vi "Lex Open Delimiter.vi"(8 "Error In":errorcluster, 11 "Lexer In":refnum<class "Lexer.lvclass">) -> (0 "Error Out":errorcluster, 3 "Lexer Out":refnum<class "Lexer.lvclass">)   [LabVIEW 2018, in "Toolkit.lvlib" / "Lexer.lvclass"]
uses:
  Lexer.lvclass
  Lexer.lvclass/Lexer.ctl
  States.ctl
  Tokens/Text/Text.lvclass
  D:/Users/cfield/Code/Field R&D Services/Labstache/src/Toolkit/Low-Level/Tokens/Token/Token.lvclass
  Tokens/Text/New.vi
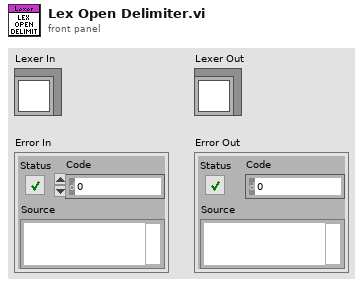
[diagram p1: front panel]
types:
  T1 = typedef "Toolkit.lvlib/Lexer.lvclass/States.ctl" = enum16{"Text", "Open Delimiter", "Tag Type", "Tag Key", "Close Delimiter"}
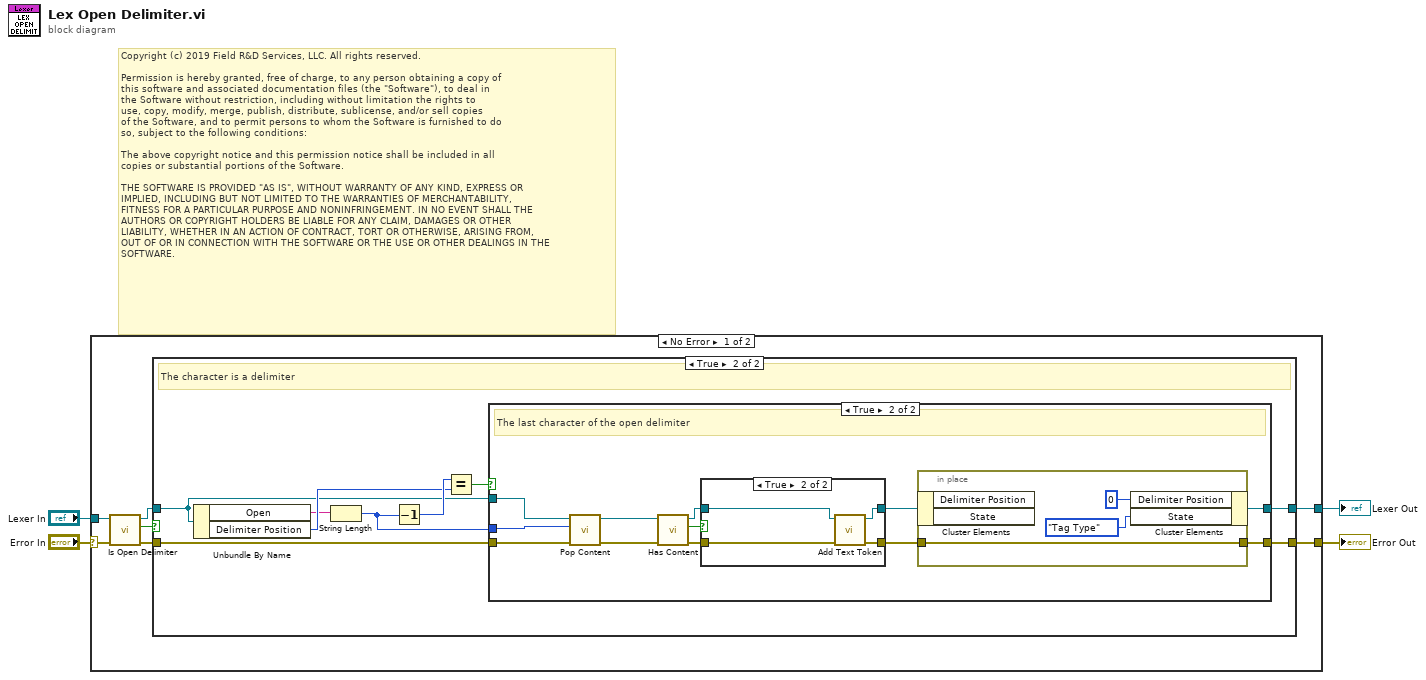
[diagram p0: block diagram]
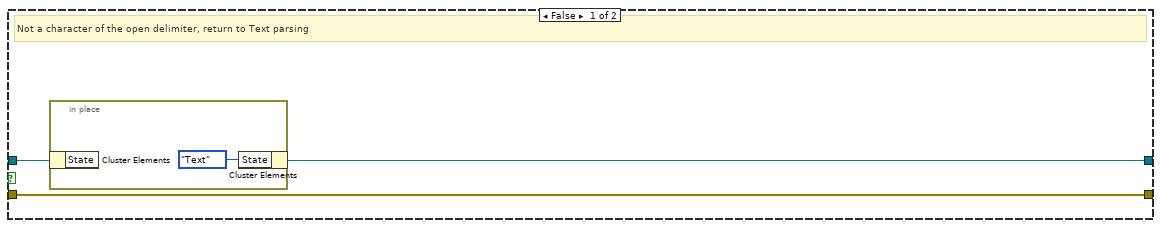
[diagram p2: hidden frame]
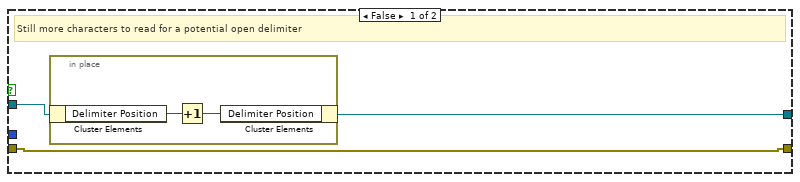
[diagram p3: hidden frame]
diagram:
  # "Copyright (c) 2019 Field R&D Services, LLC. All rights reserved.\n\nPermission is hereby granted, free of charge, to any person obtaining a copy of\nthis software and associated documentation files (the \"Software\"), to deal in\nthe Software without restriction, including without limitation the rights to\nuse, copy, modify, merge, publish, distribute, sublicense, and/or sell copies\nof the Software, and to permit persons to whom the Software is furnished to do\nso, subject to the following conditions:\n\nThe above copyright notice and this permission notice shall be included in all\ncopies or substantial portions of the Software.\n\nTHE SOFTWARE IS PROVIDED \"AS IS\", WITHOUT WARRANTY OF ANY KIND, EXPRESS OR\nIMPLIED, INCLUDING BUT NOT LIMITED TO THE WARRANTIES OF MERCHANTABILITY,\nFITNESS FOR A PARTICULAR PURPOSE AND NONINFRINGEMENT. IN NO EVENT SHALL THE\nAUTHORS OR COPYRIGHT HOLDERS BE LIABLE FOR ANY CLAIM, DAMAGES OR OTHER\nLIABILITY, WHETHER IN AN ACTION OF CONTRACT, TORT OR OTHERWISE, ARISING FROM,\nOUT OF OR IN CONNECTION WITH THE SOFTWARE OR THE USE OR OTHER DEALINGS IN THE\nSOFTWARE."
  n1 = case shown="No Error" "Error In" {
    selector: "Error In" -> [w10 w51]
    tunnel: [w6 w51] -> w4
    tunnel: [w5 w52] -> w3
    tunnel: "Lexer In" -> [w11 w52]
    frame No Error {
      n2 = call "Is Open Delimiter.vi"("Error In"=w10, "Lexer In"=w11) -> ("Error Out"=w9:errorcluster, "Open Delimiter"=w7:bool, "Lexer Out"=w8:refnum<class "Lexer.lvclass">)  [unwired: 7 in]
      n3 = case shown="True" w7 {
        tunnel: w9 -> [w14 w21]
        tunnel: w8 -> [w13 w20]
        tunnel: [w14 w18] -> w6
        tunnel: [w12 w19] -> w5
        frame False {
          # "Not a character of the open delimiter, return to Text parsing"
          n4 = in-place {
            n5 = in-place-cluster #1(w13) -> ()  [unwired: 1 out]
            n6 = in-place-cluster #1("State"=States."Text") -> (w12:refnum<class "Lexer.lvclass">)
          }
        }
        frame True {
          # "The character is a delimiter"
          n7 = Unbundle By Name(w20) -> ("Open"=w17:string, "Delimiter Position"=w23:i32)
          n8 = String Length(string=w17) -> (length=w16:i32)
          n9 = Decrement(x=w16) -> (x-1=w24:i32)
          n10 = Equal?(x=w24, y=w23) -> (x = y?=w22:bool)
          n11 = case shown="True" w22 {
            tunnel: w21 -> [w25 w40]
            tunnel: w20 -> [w27 w41]
            tunnel: [w26 w34] -> w19
            tunnel: [w25 w35] -> w18
            tunnel: w16 -> [_ w39]
            frame False {
              # "Still more characters to read for a potential open delimiter"
              n12 = in-place {
                n13 = in-place-cluster #2(w27) -> ("Delimiter Position"=w29:i32)
                n14 = Increment(x=w29) -> (x+1=w28:i32)
                n15 = in-place-cluster #2("Delimiter Position"=w28) -> (w26:refnum<class "Lexer.lvclass">)
              }
            }
            frame True {
              # "The last character of the open delimiter"
              n16 = call "Pop Content.vi"("Error In"=w40, "Characters Count"=w39, "Lexer In"=w41) -> ("Error Out"=w32:errorcluster, "Lexer Out"=w38:refnum<class "Lexer.lvclass">)  [unwired: 7 in]
              n17 = call "Has Content.vi"("Error In"=w32, "Lexer In"=w38) -> ("Error Out"=w31:errorcluster, "Content"=w30:bool, "Lexer Out"=w33:refnum<class "Lexer.lvclass">)  [unwired: 7 in]
              n18 = case shown="True" w30 {
                tunnel: [w43 w47] -> w37
                tunnel: [w42 w46] -> w36
                tunnel: w33 -> [w43 w45]
                tunnel: w31 -> [w42 w44]
                frame False {
                }
                frame True {
                  n19 = call "Add Text Token.vi"("Error In"=w44, "Lexer In"=w45) -> ("Error Out"=w46:errorcluster, "Lexer Out"=w47:refnum<class "Lexer.lvclass">)  [unwired: 8 in]
                }
              }
              n20 = in-place {
                in-place-border: w36 -> [w50]
                in-place-border: [w50] -> w35
                n21 = in-place-cluster #3(w37) -> ()  [unwired: 2 out]
                n22 = in-place-cluster #3("Delimiter Position"=0, "State"=States."Tag Type") -> (w34:refnum<class "Lexer.lvclass">)
              }
            }
          }
        }
      }
    }
    frame Error {
    }
  }
  "Error Out" <- w4
  "Lexer Out" <- w3
